vi "Monitor (1).vi"() -> (0 "error out":errorcluster, 1 "data":dbl)   [LabVIEW 2015]
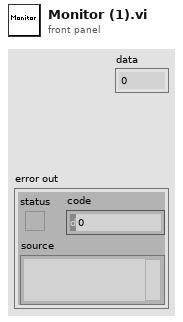
[diagram p1: front panel]
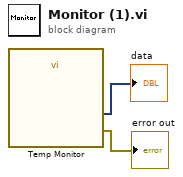
[diagram p0: block diagram]
diagram:
  n1 = call "Temp Monitor"() -> ("data"=→"data":dynamicdata, "error out"=→"error out":errorcluster)  [unwired: 17 in, 1 out]
